vi "Initialize OAuth for LinkedIn.vi"(4 "Grant Flow (PKCE)":T1, 9 "Scopes":string[](array[string])=["email", "profile", "openid"], 10 "Client Secret":string, 11 "Client ID":string) -> (3 "Oauth2.LinkedIn":refnum<class "Oauth2.LinkedIn.lvclass">)   [LabVIEW 2017, in "Oauth2.LinkedIn.lvclass"]
uses:
  Oauth2.LinkedIn.lvclass
  D:/GitHub/Oauth2/source/Oauth2/Oauth2.lvclass
  <vilib>/LabVIEW Open Source Project/OpenURI/uri/URI.lvclass
  <vilib>/LabVIEW Open Source Project/OpenURI/components/path/URI-Component.Path.lvclass
  <vilib>/LabVIEW Open Source Project/OpenURI/components/query/URI-Component.Query.lvclass
  OauthClient/OAuthClient.lvclass
  OAuthToken/OAuthAccessToken.lvclass
  Oauth2/OAuth2 Flow -- enum.ctl
  Oauth2/Oauth2.lvclass
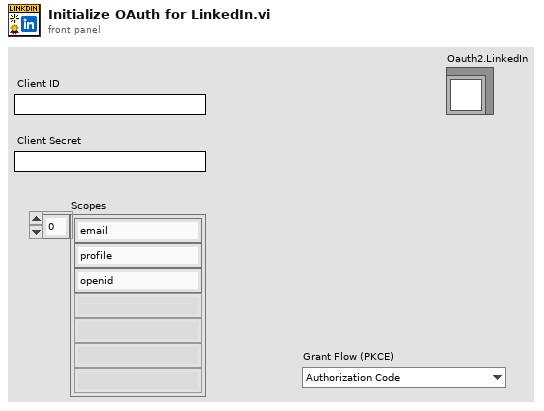
[diagram p1: front panel]
types:
  T1 = typedef "Oauth2.lvclass/OAuth2 Flow -- enum.ctl" = enum16{"Authorization Code", "Authorization Code (PKCE)", "Implicit", "Resource Owner Credentials", "Client Credentials", "Refresh Token", "Device Code"}
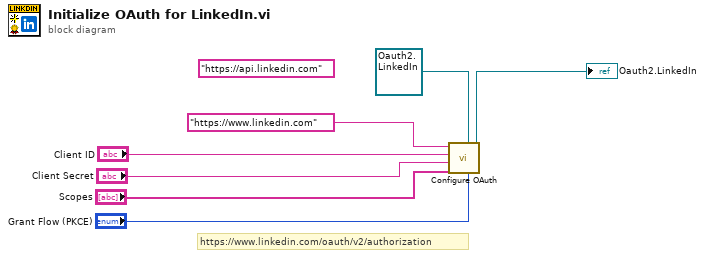
[diagram p0: block diagram]
diagram:
  (unwired) "https://api.linkedin.com" ("Authorization Server URI")
  # "https://www.linkedin.com/oauth/v2/authorization"
  n1 = call "Configure OAuth.vi"("Grant Flow (PKCE)"="Grant Flow (PKCE)", "Oauth2 in"=refnum<class "Oauth2.LinkedIn.lvclass"> refnum ("Oauth2.LinkedIn.lvclass"), "scopes"="Scopes", "Client Secret"="Client Secret", "Client ID"="Client ID", "Authorization Server URI"="https://www.linkedin.com") -> ("Oauth2"=→"Oauth2.LinkedIn":refnum<class "Oauth2.LinkedIn.lvclass">)  [unwired: 4 in, 1 out]
